vi "THERMdll.vi"(8 "error in (no error)":errorcluster, 11 "Inputs":cluster{"t":dbl, "D":dbl, "z":dbl[]}) -> (0 "error out":errorcluster, 3 "Outputs":T1)   [LabVIEW 2021]
doc: "subroutine THERMdll(t, D, z, p, e, h, s, Cv, Cp, w, hjt)\n\nCompute thermal quantities as a function of temperature, density,\nand compositions using core functions (Helmholtz free energy, ideal\ngas heat capacity and various derivatives and integrals).\n\nBased on derivations in Younglove & McLinden, JPCRD 23 #5, 1994,\nAppendix A for pressure-explicit equations (e.g. MBWR) and\nBaehr & Tillner-Roth, Thermodynamic Properties of Environmentally\nAcceptable Refrigerants, Berlin: Springer-Verlag (1995) for\nHelmholtz-explicit equations (e.g. FEQ).\n\n*** Warning *** Do NOT call this routine for two-phase states, otherwise it will return a metastable state if\nnear the phase boundary or complete nonsense at other conditions. The value of q that is returned from the flash\nroutines will indicate a two phase state by returning a value between 0 and 1. In such a situation, properties can\nonly be calculated for the saturated liquid and vapor states. For example, when calling PHFLSH: call subroutine\nPHFLSH (P,h,z,T,D,Dl,Dv,x,y,q,e,s,Cv,Cp,w,ierr,herr) If q>0 and q<1, then values of the liquid compositions\nwill be returned in the x and y arrays, and the properties of the liquid and vapor states can be calculated, for\nexample, as: call ENTRO (T,Dl,x,sliq) call ENTRO (T,Dv,x,svap)\n\nINPUTS:\nt --temperature [K]\nD --molar density [mol/L]\nz --composition [array of mol frac]\n\nOUTPUTS:\np --pressure [kPa]\ne --internal energy [J/mol]\nh --enthalpy [J/mol]\ns --entropy [J/mol-K]\nCv --isochoric heat capacity [J/mol-K]\nCp --isobaric heat capacity [J/mol-K]\nw --speed of sound [m/s]\nhjt --isenthalpic Joule-Thomson coefficient [K/kPa]"
uses:
  REFPROP.dll
panel:
  # "REFPROP-THERMdll.vi"
  # "void  THERMdll(double *t, double *D, double *z, double *p, double *e, double *h, double *s, double *Cv, double *Cp, double *w, double *hjt)"
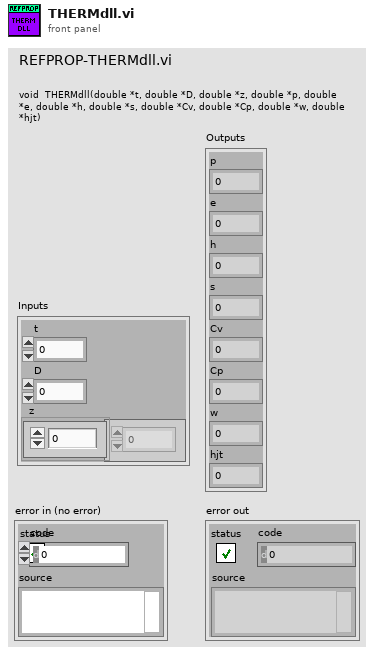
[diagram p1: front panel]
types:
  T1 = cluster{"p":dbl, "e":dbl, "h":dbl, "s":dbl, "Cv":dbl, "Cp":dbl, "w":dbl, "hjt":dbl}
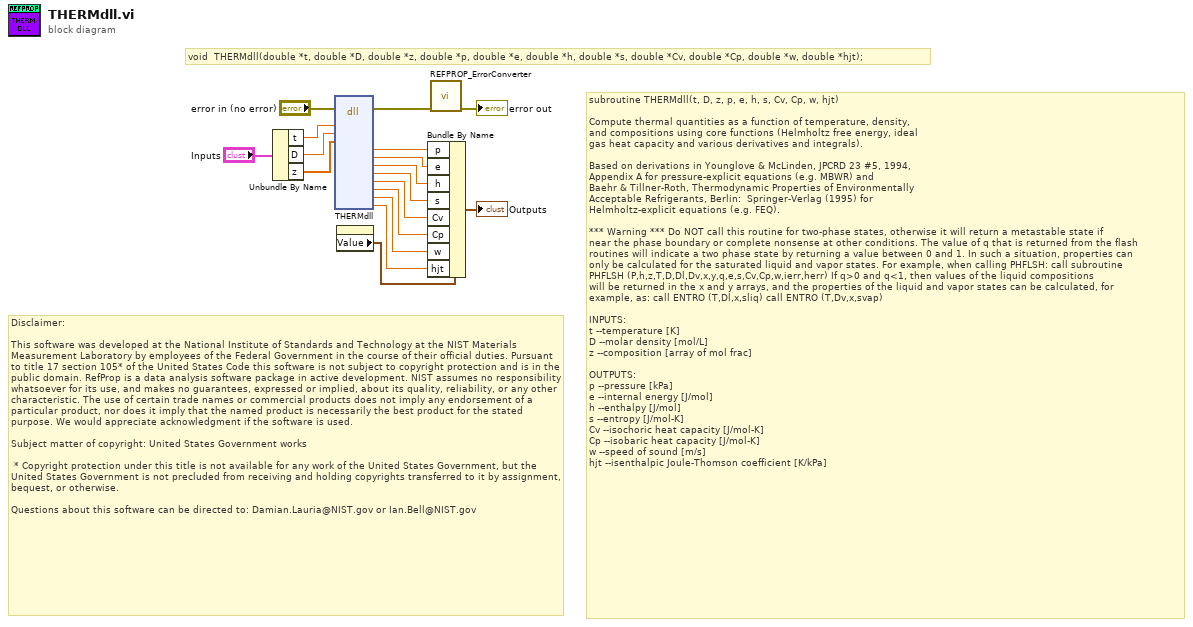
[diagram p0: block diagram]
diagram:
  # "Disclaimer:\n\nThis software was developed at the National Institute of Standards and Technology at the NIST Materials Measurement Laboratory by employees of the Federal Government in the course of their official duties. Pursuant to title 17 section 105* of the United States Code this software is not subject to copyright protection and is in the public domain. RefProp is a data analysis software package in active development. NIST assumes no responsibility whatsoever for its use, and makes no guarantees, expressed or implied, about its quality, reliability, or any other characteristic. The use of certain trade names or commercial products does not imply any endorsement of a particular product, nor does it imply that the named product is necessarily the best product for the stated purpose. We would appreciate acknowledgment if the software is used.\n \nSubject matter of copyright: United States Government works\n  \n * Copyright protection under this title is not available for any work of the United States Government, but the United States Government is not precluded from receiving and holding copyrights transferred to it by assignment, bequest, or otherwise.\n\nQuestions about this software can be directed to: Damian.Lauria@NIST.gov or Ian.Bell@NIST.gov"
  # "void  THERMdll(double *t, double *D, double *z, double *p, double *e, double *h, double *s, double *Cv, double *Cp, double *w, double *hjt);"
  # "subroutine THERMdll(t, D, z, p, e, h, s, Cv, Cp, w, hjt)\n\nCompute thermal quantities as a function of temperature, density,\nand compositions using core functions (Helmholtz free energy, ideal\ngas heat capacity and various derivatives and integrals).\n\nBased on derivations in Younglove & McLinden, JPCRD 23 #5, 1994,\nAppendix A for pressure-explicit equations (e.g. MBWR) and\nBaehr & Tillner-Roth, Thermodynamic Properties of Environmentally\nAcceptable Refrigerants, Berlin:  Springer-Verlag (1995) for\nHelmholtz-explicit equations (e.g. FEQ).\n\n*** Warning *** Do NOT call this routine for two-phase states, otherwise it will return a metastable state if\nnear the phase boundary or complete nonsense at other conditions. The value of q that is returned from the flash\nroutines will indicate a two phase state by returning a value between 0 and 1. In such a situation, properties can\nonly be calculated for the saturated liquid and vapor states. For example, when calling PHFLSH: call subroutine\nPHFLSH (P,h,z,T,D,Dl,Dv,x,y,q,e,s,Cv,Cp,w,ierr,herr) If q>0 and q<1, then values of the liquid compositions\nwill be returned in the x and y arrays, and the properties of the liquid and vapor states can be calculated, for\nexample, as: call ENTRO (T,Dl,x,sliq) call ENTRO (T,Dv,x,svap)\n\nINPUTS:\nt --temperature [K]\nD --molar density [mol/L]\nz --composition [array of mol frac]\n\nOUTPUTS:\np --pressure [kPa]\ne --internal energy [J/mol]\nh --enthalpy [J/mol]\ns --entropy [J/mol-K]\nCv --isochoric heat capacity [J/mol-K]\nCp --isobaric heat capacity [J/mol-K]\nw --speed of sound [m/s]\nhjt --isenthalpic Joule-Thomson coefficient [K/kPa]"
  n1 = Unbundle By Name("Inputs") -> ("t"=w13:dbl, "D"=w12:dbl, "z"=w11:dbl[])
  n2 = dll-call lib="C:/Users/lauria/OneDrive - National Institute of Standards and Technology (NIST)/LabVIEW Projects/7 REFPROP/REFPROP-wrappers-master/REFPROP-wrappers-master/wrappers/Labview/REFPROP/REFPROP.*" fn="THERMdll"(error in="error in (no error)", "t"=w13, "D"=w12, "z"=w11) -> (error out=w17:errorcluster, "p"=w1:dbl, "e"=w2:dbl, "h"=w3:dbl, "s"=w4:dbl, "Cv"=w5:dbl, "Cp"=w6:dbl, "w"=w7:dbl, "hjt"=w8:dbl)  [unwired: 14 in, 1 out]
  n3 = property on="Outputs" class="Clust (strict)"() -> ("Value"=w9:T1)  [unwired: 2 in, 2 out]
  n4 = Bundle By Name(cluster=w9, "p"=w1, "e"=w2, "h"=w3, "s"=w4, "Cv"=w5, "Cp"=w6, "w"=w7, "hjt"=w8) -> (→"Outputs":T1)
  n5 = call "REFPROP_ErrorConverter.vi"("error in (no error)"=w17) -> ("error out"=→"error out":errorcluster)  [unwired: 10 in]
